vi "Touch VISA Global.vi"() -> ()   [LabVIEW 2025]
panel:
  out "Touch VISA Global":refnum<visa-resource-name>
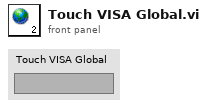
[diagram p1: front panel]
diagram:
